vi "Scale Progress Bar Range.vi"(9 "Value":dbl, 10 "Minimum":dbl, 11 "Maximum":dbl) -> (1 "Value Out":dbl, 3 "Maximum Out":dbl)   [LabVIEW 2015, in "Front Panel Publisher.lvlib" / "Progressbar.lvclass"]
uses:
  Progressbar.lvclass
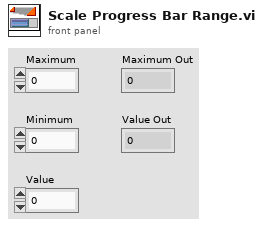
[diagram p1: front panel]
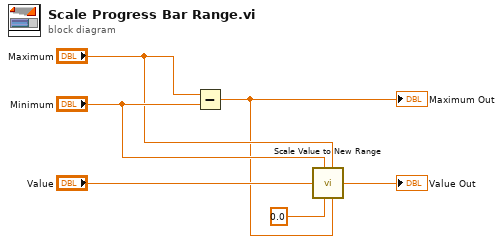
[diagram p0: block diagram]
diagram:
  n1 = Subtract(x="Maximum", y="Minimum") -> (x-y=w2:dbl)
  "Maximum Out" <- w2
  n2 = call <vilib>:"Scale Value to New Range.vi"("original minimum"="Minimum", "original value"="Value", "new minimum"=0.0, "original maximum"="Maximum", "new maximum"=w2) -> ("scaled value"=→"Value Out":dbl)  [unwired: 4 in]
